vi "sv_Prepare Data for Resampling (Time to Angle).vi"(11 "Array":waveform(dbl)[](array[waveform])) -> (0 "channel count":i32, 1 "signal len":i32, 2 "fs":dbl format="%.2f", 3 "Y":dbl[](array[numeric]) format="%.2f", 5 "elapsed length":dbl)   [LabVIEW 2017, in "SoundVib_ContSweptSine.lvlib"]
uses:
  <vilib>/addons/Sound and Vibration/svt_Continuous Swept Sine/SoundVib_ContSweptSine.lvlib
  <vilib>/Waveform/WDTOps.llb/WDT Number of Waveform Samples DBL.vi
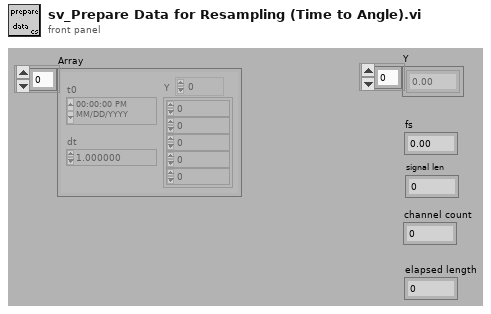
[diagram p1: front panel]
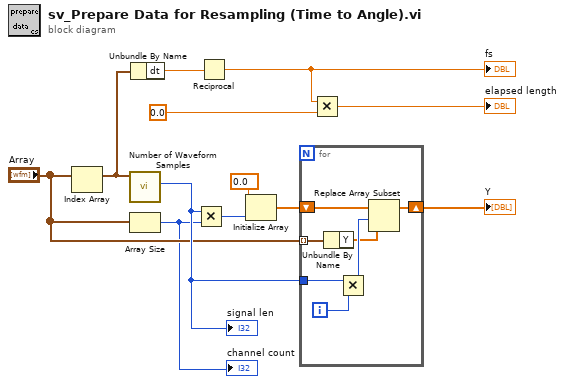
[diagram p0: block diagram]
diagram:
  n1 = Index Array(array="Array") -> (element=w4:waveform(dbl))  [unwired: 1 in]
  n2 = call-poly <vilib>:"Number of Waveform Samples.vi"("waveform in"=w4) -> ("number of samples"=w9:i32)  [unwired: 8 in, 2 out]
  "signal len" <- w9
  n3 = Array Size(array="Array") -> (size(s)=w5:i32)
  "channel count" <- w5
  n4 = Unbundle By Name(w4) -> ("dt"=w6:dbl)
  n5 = Multiply(x=w9, y=w5) -> (x*y=w12:i32)
  n6 = Reciprocal(x=w6) -> (1/x=w2:dbl)
  "fs" <- w2
  n7 = Initialize Array(0.0 ("element"), w12) -> (w10:dbl[])
  n8 = for {
    shift-right: [w13] -> w7
    shift-left: w10 -> [w19]
    tunnel: w9 -> [w17]
    tunnel: "Array" -> [w15] mode=indexing
    i -> [w18]
    n9 = Unbundle By Name(w15) -> ("Y"=w14:dbl[])
    n10 = Multiply(x=w17, y=w18) -> (x*y=w16:i32)
    n11 = Replace Array Subset(array=w19, new element=w14, index=w16) -> (w13:dbl[])
  }
  "Y" <- w7
  n12 = Multiply(x=w2, y=0.0) -> (x*y=→"elapsed length":dbl)
